vi "Move motor--subVI.vi"(8 "error in (no error)":errorcluster, 10 "Motor params":T1={"Motor type"=enum."Unipolar", "Direction"=enum."CW", "Steps"=1000, "Frequency (Hz)"=20, "Step type"=enum."Full"}, 11 "VISA Refnum in":refnum<visa-resource-name>) -> (0 "error out":errorcluster, 2 "Data read":string, 3 "Data written":string)   [LabVIEW 2020, in "Arduino stepper.lvlib"]
uses:
  Arduino stepper.lvlib
  Motor parameters.ctl
  <vilib>/Instr/_visa.llb/VISA Flush IO Buffer Mask.ctl
panel:
  out "concatenated string":string
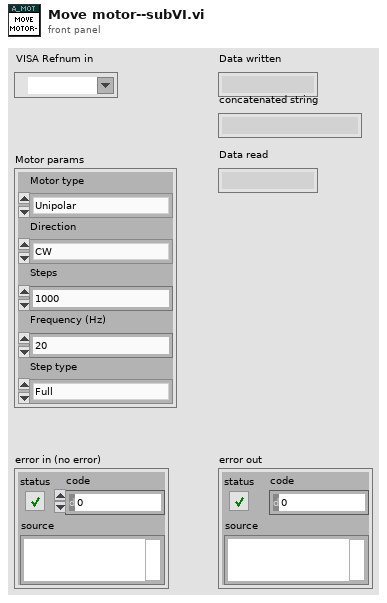
[diagram p1: front panel]
types:
  T1 = typedef "Arduino stepper.lvlib/Motor parameters.ctl" = cluster{"Motor type":enum8{"", "Unipolar", "Bipolar"}, "Direction":enum8{"", "CW", "CCW"}, "Steps":u16, "Frequency (Hz)":u8, "Step type":enum8{"", "Half", "Full"}}
  T2 = typedef "VISA Flush IO Buffer Mask.ctl" = u16
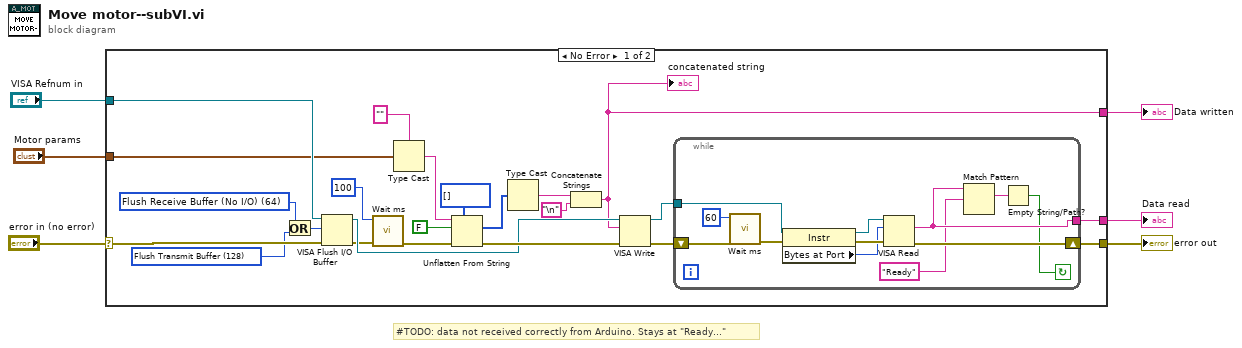
[diagram p0: block diagram]
diagram:
  # "#TODO: data not received correctly from Arduino. Stays at \"Ready...\""
  n1 = case shown="No Error" "error in (no error)" {
    selector: "error in (no error)" -> [w16 w42]
    tunnel: [w12 w42] -> w6
    tunnel: "VISA Refnum in" -> [w17 _]
    tunnel: "Motor params" -> [w15 _]
    tunnel: [w14 _] -> w2
    tunnel: [w10 _] -> w1
    frame No Error {
      w8 = T2 64 items=["Flush Receive Buffer"=16, "Write Transmit Buffer to Device"=32, "Flush Receive Buffer (No I/O)"=64, "Flush Transmit Buffer"=128] ("Mask")
      w7 = T2 128 items=["Flush Receive Buffer"=16, "Write Transmit Buffer to Device"=32, "Flush Receive Buffer (No I/O)"=64, "Flush Transmit Buffer"=128] ("Mask")
      n2 = Or(x=w8, y=w7) -> (x .or. y?=w9:T2)
      n3 = VISA Flush I/O Buffer(VISA resource name=w17, mask (16)=w9, error in (no error)=w16) -> (VISA resource name out=w20:refnum<visa-resource-name>, error out=w18:errorcluster)
      n4 = call "Wait ms.vi"("error in (no error)"=w18, "milliseconds to wait"=u32 100) -> ("error out"=w22:errorcluster)  [unwired: 9 in]
      n5 = Type Cast(type="", x=w15) -> (*(type *) &x=w24:string)
      n6 = Unflatten From String(type=u8[] [], binary string=w24, data includes array or string size? (T)=FALSE ("prepend array or string size? (T)"), error in (no error)=w22) -> (value=w27:u8[], error out=w23:errorcluster)  [unwired: 1 in, 1 out]
      n7 = Type Cast(x=w27) -> (*(type *) &x=w28:string)  [unwired: 1 in]
      n8 = Concatenate Strings(w28, "\n") -> (w14:string)
      "concatenated string" <- w14
      n9 = VISA Write(VISA resource name=w20, write buffer=w14, error in (no error)=w23) -> (VISA resource name out=w11:refnum<visa-resource-name>, error out=w13:errorcluster)  [unwired: 1 out]
      n10 = while {
        tunnel: w11 -> [w36]
        tunnel: [w33] -> w10
        shift-right: [w39] -> w12
        shift-left: w13 -> [w41]
        stop <- w30 continue-if-true
        n11 = call "Wait ms.vi"("error in (no error)"=w41, "milliseconds to wait"=u32 60) -> ("error out"=w38:errorcluster)  [unwired: 9 in]
        n12 = property class="Instr"(reference=w36, error in=w38) -> (reference out=w35:refnum<visa-resource-name>, error out=w37:errorcluster, "Bytes at Port"=w34:u32)
        n13 = VISA Read(VISA resource name=w35, byte count=w34, error in (no error)=w37) -> (read buffer=w33:string, error out=w39:errorcluster)  [unwired: 2 out]
        n14 = Match Pattern(string=w33, regular expression="Ready" ("y")) -> (match substring=w31:string)  [unwired: 1 in, 3 out]
        n15 = Empty String/Path?(string/path=w31) -> (empty?=w30:bool)
      }
    }
    frame Error {
    }
  }
  "error out" <- w6
  "Data written" <- w2
  "Data read" <- w1
